vi "Current Reading and Storing.vi"() -> ()   [LabVIEW 2012]
uses:
  <vilib>/Utility/file.llb/Write To Spreadsheet File (string).vi
panel:
  out "Current":dbl format="%^.2e"
  in  "resource name (don't change)":string="KE6485ExampleInstr"
  in  "stop":bool
  in  "file path (dialog if empty)":path
  # "Reading Current and Storing Current in Excel File"
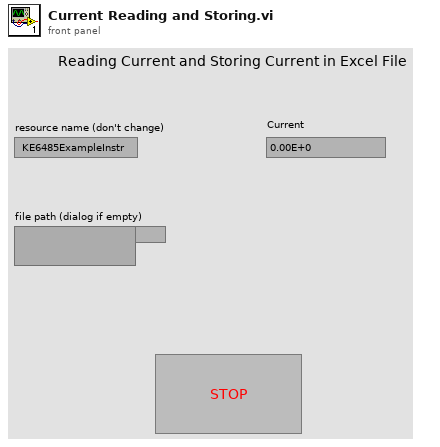
[diagram p1: front panel]
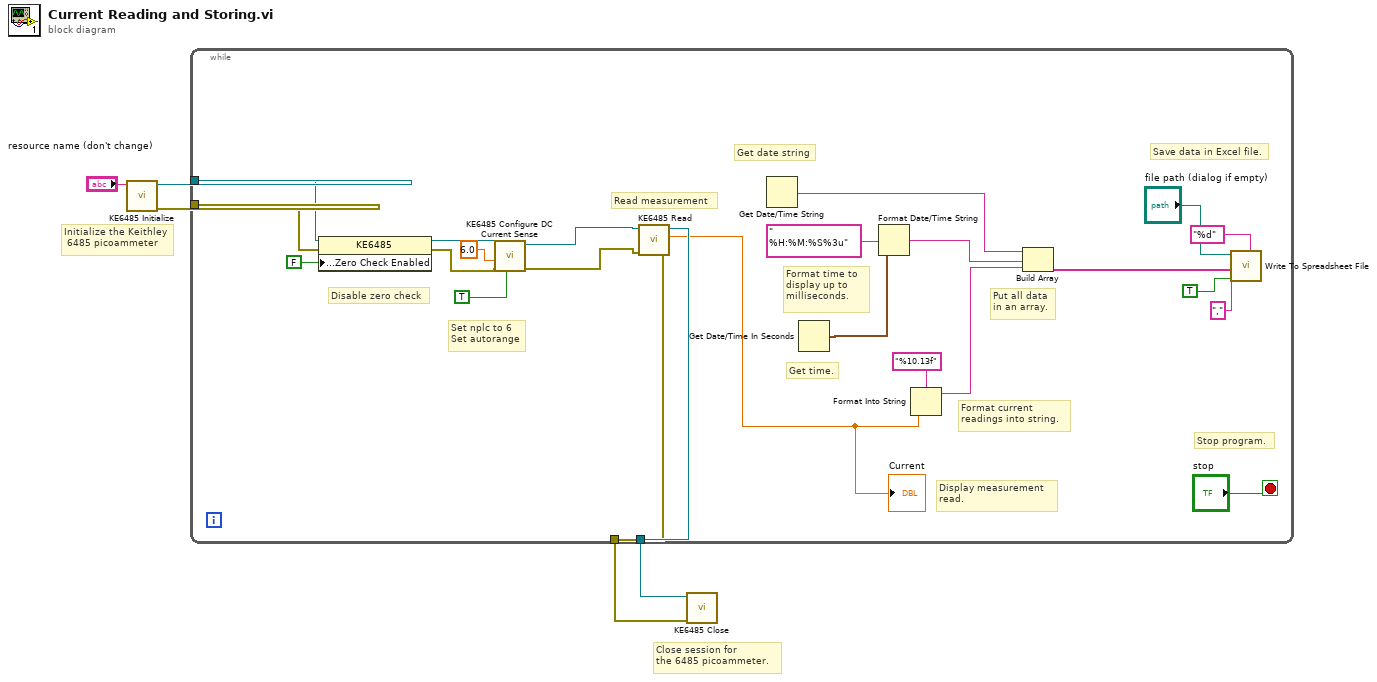
[diagram p0: block diagram]
diagram:
  # "Close session for \nthe 6485 picoammeter."
  # "Initialize the Keithley\n 6485 picoammeter"
  n1 = call <instrlib>:"KE6485 Initialize.vi"("resource name"="resource name (don't change)") -> ("error out"=w1:errorcluster, "instrument handle out"=w2:refnum<k15>)  [unwired: 9 in]
  n2 = while {
    tunnel: w2 -> [w18]
    tunnel: [w29] -> w5
    tunnel: w1 -> [w16]
    tunnel: [w28] -> w4
    stop <- "stop" stop-if-true
    # "Format current \nreadings into string."
    # "Save data in Excel file."
    # "Stop program."
    # "Put all data\nin an array."
    # "Format time to \ndisplay up to\nmilliseconds."
    # "Get time."
    # "Display measurement \nread."
    # "Get date string"
    # "Read measurement"
    # "Set nplc to 6\nSet autorange"
    # "Disable zero check"
    n3 = property class="KE6485"(reference=w18, error in=w16, "System Settings:Zero Check Enabled"=FALSE) -> (reference out=w14:refnum<k15>, error out=w13:errorcluster)
    n4 = call <instrlib>:"KE6485 Configure DC Current Sense.vi"("autorange"=TRUE, "error in (no error)"=w13, "nplc"=6.0, "instrument handle"=w14) -> ("error out"=w12:errorcluster, "instrument handle out"=w11:refnum<k15>)  [unwired: 6 in]
    n5 = call <instrlib>:"KE6485 Read.vi"("error in (no error)"=w12, "instrument handle"=w11) -> ("error out"=w28:errorcluster, "reading"=w15:dbl, "instrument handle out"=w29:refnum<k15>)  [unwired: 7 in]
    "Current" <- w15
    n6 = Get Date/Time String() -> (date string=w8:string)  [unwired: 3 in, 1 out]
    n7 = Get Date/Time In Seconds() -> (seconds since 1Jan1904=w6:timestamp)
    n8 = Format Date/Time String(time format string (%c)="            %H:%M:%S%3u", seconds (now)=w6) -> (date/time string=w7:string)  [unwired: 1 in]
    n9 = Format Into String(format string="%10.13f", w15) -> (resulting string=w27:string)  [unwired: 2 in, 1 out]
    n10 = Build Array(w8, w7, w27) -> (w26:string[])
    n11 = call-poly <vilib>:"Write To Spreadsheet File.vi"("delimiter (\\t)"="," ("delimiter (\\t)"), "format (%s)"="%d", "append to file? (new file:F)"=TRUE, "1D data"=w26, "file path (dialog if empty)"="file path (dialog if empty)") -> ()  [unwired: 3 in, 1 out]
  }
  n12 = call <instrlib>:"KE6485 Close.vi"("error in (no error)"=w4, "instrument handle"=w5) -> ()  [unwired: 9 in, 1 out]
